vi "calcF.vi"(8 "error in (no error)":errorcluster, 9 "Matrix H":dbl[][](array[numeric]), 10 "Q Matrix":dbl[][](array[numeric]), 11 "OptCtrl in":refnum<class "OptCtrl.lvclass">) -> (0 "error out":errorcluster, 2 "F Matrix":dbl[][](array[numeric]), 3 "OptCtrl out":refnum<class "OptCtrl.lvclass">)   [LabVIEW 2016, in "OptCtrl.lvclass"]
doc: "Calculate the F matrix. F = inv(A.T * C.T * C * A + rho * H)."
uses:
  OptCtrl.lvclass
  <vilib>/Analysis/baseanly.llb/Matrix Type of Inverse Matrix.ctl
  OptCtrl.lvclass/OptCtrl.ctl
  <vilib>/Analysis/Matrix/Numeric/Conversions/Array To Matrix - RA2.vi
  <vilib>/Analysis/baseanly.llb/Real Inverse Matrix.vi
  <vilib>/Analysis/Matrix/Numeric/Conversions/Matrix To Array - RM.vi
  <vilib>/Analysis/Matrix/NI_Matrix.lvlib
  <vilib>/Analysis/NI_AALBase.lvlib
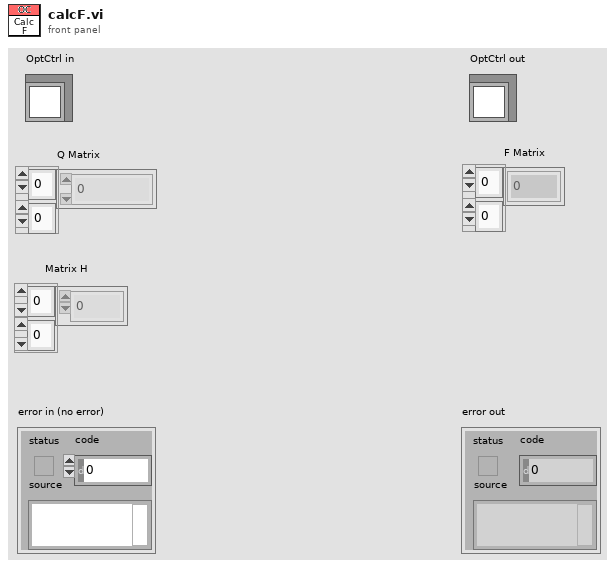
[diagram p1: front panel]
types:
  T1 = typedef "NI_AALBase.lvlib/Matrix Type of Inverse Matrix.ctl" = enum32{"General", "Positive Definite", "Lower Triangular", "Upper Triangular"}
  T2 = typedef "NI_Matrix.lvlib/RealMatrix.ctl" = dbl[][]
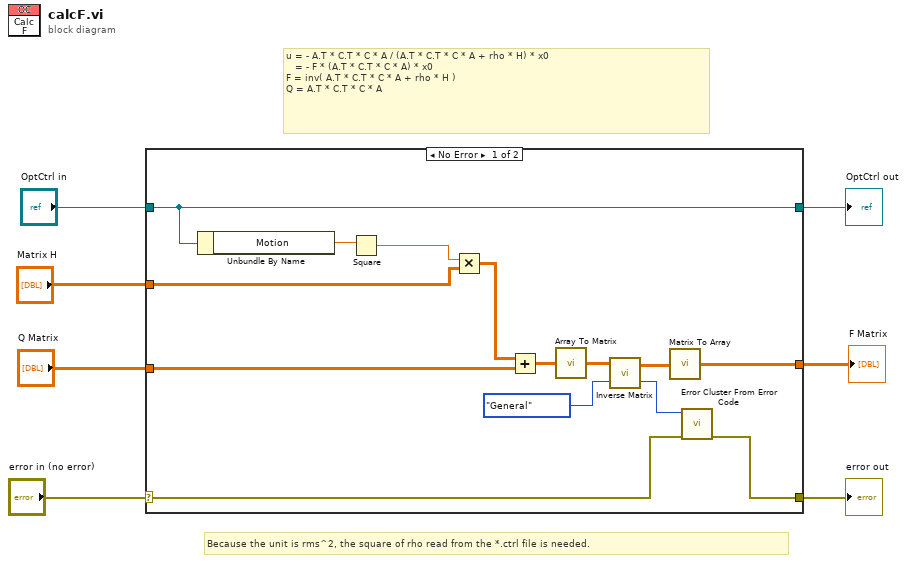
[diagram p0: block diagram]
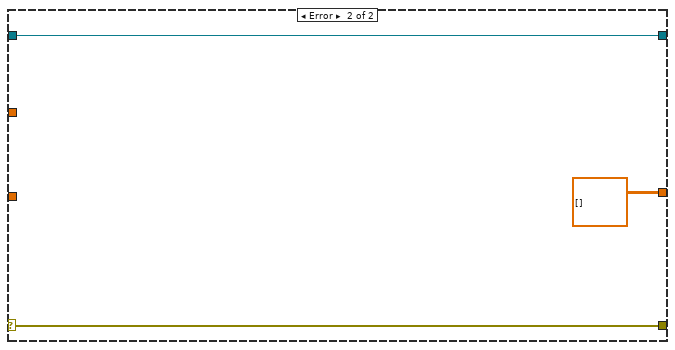
[diagram p2: hidden frame]
diagram:
  # "Because the unit is rms^2, the square of rho read from the *.ctrl file is needed."
  # "u = - A.T * C.T * C * A / (A.T * C.T * C * A + rho * H) * x0\n   = - F * (A.T * C.T * C * A) * x0\nF = inv( A.T * C.T * C * A + rho * H )\nQ = A.T * C.T * C * A"
  n1 = case shown="No Error" "error in (no error)" {
    selector: "error in (no error)" -> [w10 w24]
    tunnel: [w16 w24] -> w6
    tunnel: [w9 w23] -> w4
    tunnel: "OptCtrl in" -> [w9 w23]
    tunnel: "Q Matrix" -> [w18 _]
    tunnel: "Matrix H" -> [w11 _]
    tunnel: [w8 dbl[][] [] ("Real 2D Array")] -> w1
    frame No Error {
      n2 = Unbundle By Name(w9) -> ("Motion"=w21:dbl)
      n3 = Square(x=w21) -> (x^2=w20:dbl)
      n4 = Multiply(x=w20, y=w11) -> (x*y=w19:dbl[][])
      n5 = Add(x=w19, y=w18) -> (x+y=w14:dbl[][])
      n6 = call-poly <vilib>:"Array To Matrix.vi"("Real 2D Array"=w14) -> ("Real Matrix"=w13:T2)
      n7 = call-poly <vilib>:"Inverse Matrix.vi"("matrix type"=Matrix_Type_of_Inverse_Matrix."General", "Input Matrix"=w13) -> ("error"=w17:i32, "Inverse Matrix"=w15:T2)
      n8 = call-poly <vilib>:"Matrix To Array.vi"("Real Matrix"=w15) -> ("Real 2D Array"=w8:dbl[][])
      n9 = call <vilib>:"Error Cluster From Error Code.vi"("error in (no error)"=w10, "error code (0)"=w17) -> ("error out"=w16:errorcluster)  [unwired: 7 in]
    }
    frame Error {
    }
  }
  "error out" <- w6
  "OptCtrl out" <- w4
  "F Matrix" <- w1
